vi "Change Laser Enable State.vi"(8 "error in":errorcluster, 11 "cPAS in":refnum<class "cPAS.lvclass">) -> (0 "error out":errorcluster, 3 "cPAS out":refnum<class "cPAS.lvclass">)   [LabVIEW 2015, in "cPAS.lvclass"]
uses:
  cPAS.lvclass
  cPAS.lvclass/cPAS.ctl
  <vilib>/Utility/error.llb/Error Cluster From Error Code.vi
  <vilib>/rvi/errors/niLvFpgaAdjustHostInterfaceError.vi
  <vilib>/rvi/interface/nirviReadWriteControl/nirviReadWriteControl.xnode
  Interface/fpga_ctl.ctl
  FPGA Bitfiles/FPGA Server.lvbitx
  Reusable/Instrument/Instrument.lvclass
  NiFpgaLv.dll
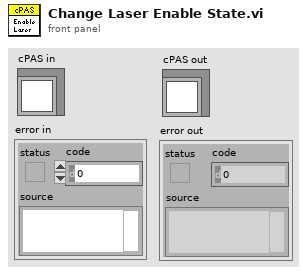
[diagram p1: front panel]
types:
  T1 = typedef "fpga_ctl.ctl" = refnum<k20>
  T2 = cluster{"Array of Boolean[0]":bool, "Array of Boolean[1]":bool, "Array of Boolean[2]":bool, "Array of Boolean[3]":bool, "Array of Boolean[4]":bool}
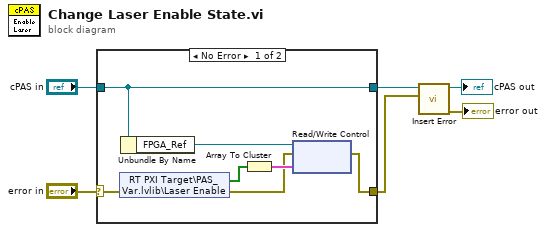
[diagram p0: block diagram]
diagram:
  n1 = case shown="No Error" "error in" {
    selector: "error in" -> [w10 w15]
    tunnel: [w11 w15] -> w2
    tunnel: [w13 w14] -> w4
    tunnel: "cPAS in" -> [w13 w14]
    frame No Error {
      n2 = shared-variable "RT PXI Target\\PAS_Var.lvlib\\Laser Enable"(error in=w10) -> (w9:bool[], error out=w7:errorcluster)
      n3 = Unbundle By Name(w13) -> ("FPGA_Ref"=w12:T1)
      n4 = Array To Cluster(array=w9) -> (cluster=w8:T2)
      n5 = xnode "Read/Write Control"("FPGA VI Reference In"=w12, "error in"=w7, "LaserEn"=w8) -> ("error out"=w11:errorcluster)  [unwired: 1 out]
    }
    frame Error {
    }
  }
  n6 = call "Insert Error.vi"("err"=w2, "Instrument in"=w4) -> ("error out"=→"error out":errorcluster, "Instrument out"=→"cPAS out":refnum<class "cPAS.lvclass">)  [unwired: 7 in, 1 out]
